vi "万能延时模块.vi"(6 "等待时间（50ms）":u32=50, 8 "错误输入":errorcluster, 11 "in":variant) -> (0 "错误输出":errorcluster caption="错误输入", 3 "out":variant)   [LabVIEW 2013]
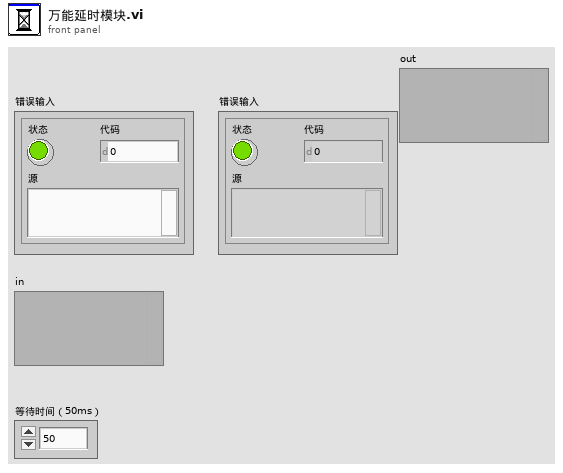
[diagram p1: front panel]
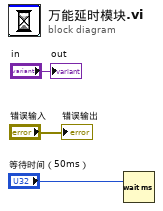
[diagram p0: block diagram]
diagram:
  n1 = Wait (ms)(milliseconds to wait="等待时间（50ms）") -> ()  [unwired: 1 out]
  "错误输出" <- "错误输入"
  "out" <- "in"
